vi "Initialize.vi"(8 "error in":errorcluster, 10 "Plugin Name":string, 11 "Resistance Control in":refnum<class "Resistance Control.lvclass">) -> (0 "error out":errorcluster, 3 "Resistance Control out":refnum<class "Resistance Control.lvclass">)   [LabVIEW 2023, in "Resistance Control.lvclass"]
uses:
  Resistance Control.lvclass
  Resistance Control.lvclass/Resistance Control.ctl
  <vilib>/ADAS Replay HIL/Channels/Tag Wrapper/Polymorphic/Open Producer Tag (Double).vi
  <vilib>/ADAS Replay HIL/Channels/Tag Wrapper/Polymorphic/Open Consumer Tag (Double).vi
  <vilib>/ADAS Replay HIL/Channels/Tag Wrapper/Polymorphic/Open Producer Tag (Double).vi/45cd6eaa-a1ce-41a4-8aba-62a49d103d7e.vi
  <vilib>/ADAS Replay HIL/Channels/Tag Wrapper/Polymorphic/Open Consumer Tag (Double).vi/bacb721e-673a-491a-accd-959f2e1f334e.vi
  <vilib>/ADAS Replay HIL/Channels/Tag Wrapper/Polymorphic/Open Producer Tag (Double).vi/45cd6eaa-a1ce-41a4-8aba-62a49d103d7e.vi/c28b0ead-42ad-4072-80a2-aca7f2bd7ce3.vi
  <vilib>/ADAS Replay HIL/Channels/Tag Wrapper/Polymorphic/Open Consumer Tag (Double).vi/bacb721e-673a-491a-accd-959f2e1f334e.vi/c28b0ead-42ad-4072-80a2-aca7f2bd7ce3.vi
  <vilib>/ADAS Replay HIL/AdasHilServices/AdasHilServices Fill In Error Info Ex.vi
  <vilib>/ADAS Replay HIL/Channels/Tag Wrapper/Tag Wrapper.lvlib
  Capability/Capability.lvclass
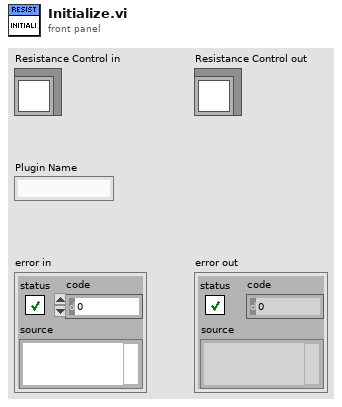
[diagram p1: front panel]
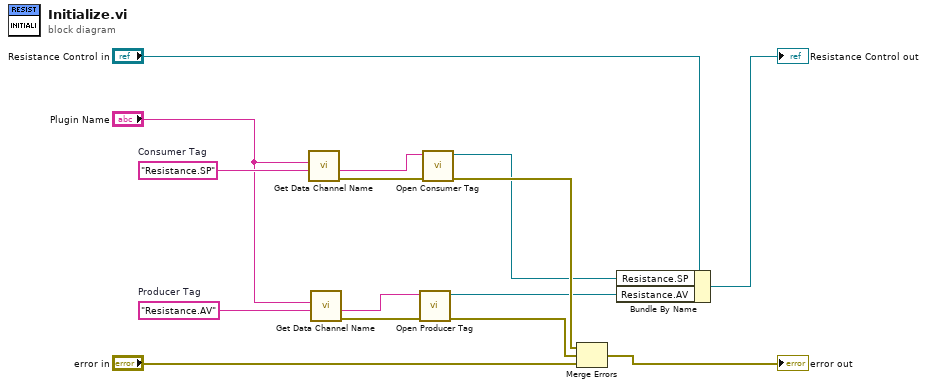
[diagram p0: block diagram]
diagram:
  w11 = "Resistance.AV"  # Producer Tag
  w15 = "Resistance.SP"  # Consumer Tag
  n1 = call "Get Data Channel Name.vi"("Channel Name"=w15, "Plugin Name"="Plugin Name") -> ("error out"=w10:errorcluster, "Data Channel Name"=w14:string)  [unwired: 8 in]
  n2 = call "Get Data Channel Name.vi"("Channel Name"=w11, "Plugin Name"="Plugin Name") -> ("error out"=w9:errorcluster, "Data Channel Name"=w12:string)  [unwired: 8 in]
  n3 = call-poly <vilib>:"Open Producer Tag.vi"("error in"=w9, "Channel Name"=w12) -> ("error out"=w5:errorcluster, "ADAS HIL Channel"=w1:refnum<k21>)  [unwired: 8 in]
  n4 = call-poly <vilib>:"Open Consumer Tag.vi"("error in"=w10, "Channel Name"=w14) -> ("error out"=w6:errorcluster, "ADAS HIL Channel"=w2:refnum<k21>)  [unwired: 8 in]
  n5 = Merge Errors(w6, w5, "error in") -> (→"error out":errorcluster)
  n6 = Bundle By Name(cluster="Resistance Control in", "Resistance.SP"=w2, "Resistance.AV"=w1) -> (→"Resistance Control out":refnum<class "Resistance Control.lvclass">)
